vi "Mean Signal.vi"(7 "initialize":bool, 9 "sample length":i32=10, 11 "Signal In":dbl format="%0.2f") -> (3 "Signal Out":dbl format="%0.2f")   [LabVIEW 2011]
uses:
  <vilib>/ptbypt/NI_PtbyPt.lvlib
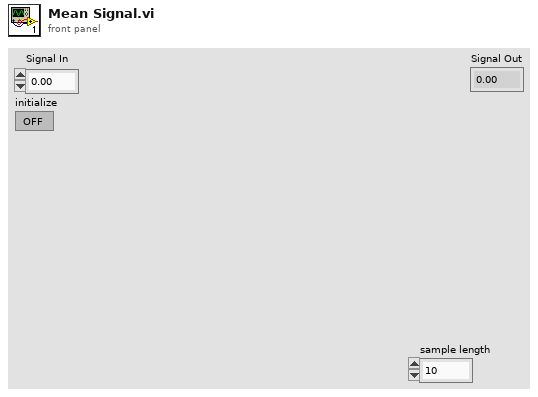
[diagram p1: front panel]
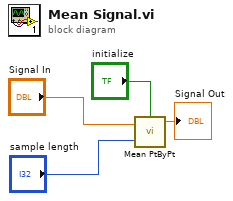
[diagram p0: block diagram]
diagram:
  n1 = call <vilib>:"Mean PtByPt.vi"("x"="Signal In", "sample length"="sample length", "initialize"="initialize") -> ("mean"=→"Signal Out":dbl)  [unwired: 1 in, 1 out]
